vi "CheckVirtualSetup.vi"(8 "error in (no error)":errorcluster, 11 "VirtualDataTable":string[](array[string])) -> (0 "error out":errorcluster, 2 "VirtualNames":cluster{string[]}[](array[cluster]), 3 "VirtualSetups":string[](array[string]))   [LabVIEW 2014, in "Project.lvclass"]
uses:
  Project.lvclass
  VirtualSetupDataTypeDefine.ctl
  Virtual/Control/AllVirtualTypeData.ctl
  Virtual/VirtualOrigin.lvclass
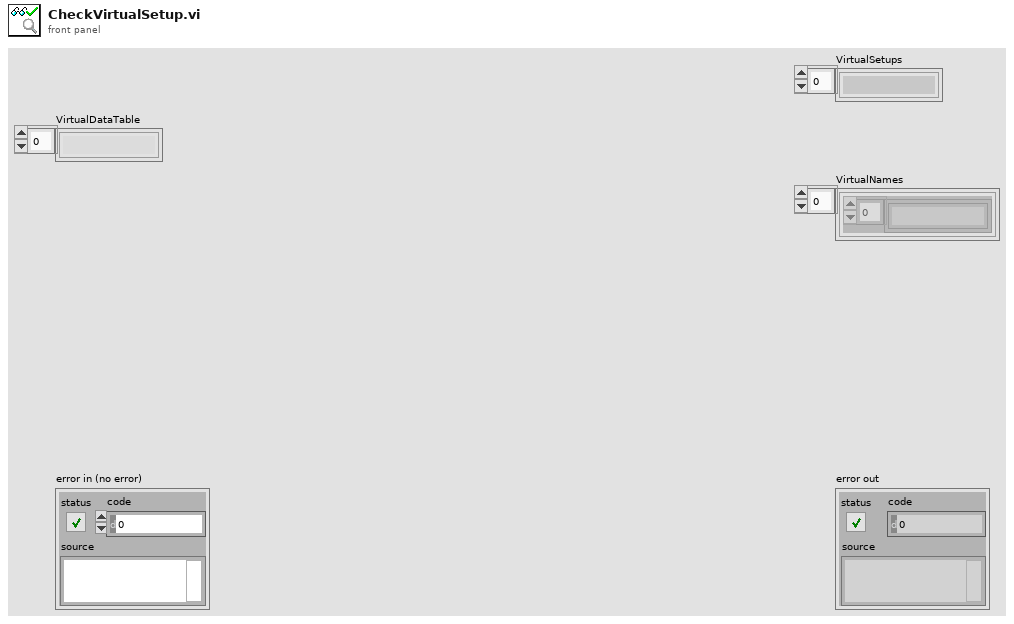
[diagram p1: front panel]
types:
  T1 = typedef "Project.lvclass/VirtualSetupDataTypeDefine.ctl" = T2[]
  T2 = typedef "VirtualOrigin.lvclass/AllVirtualTypeData.ctl" = cluster{"Search Name":string, "Start X":dbl, "Increase X":dbl, "X Step":i32, "Start Y":dbl, "Increase Y":dbl, "Y Step":i32, "Sensor":i32}
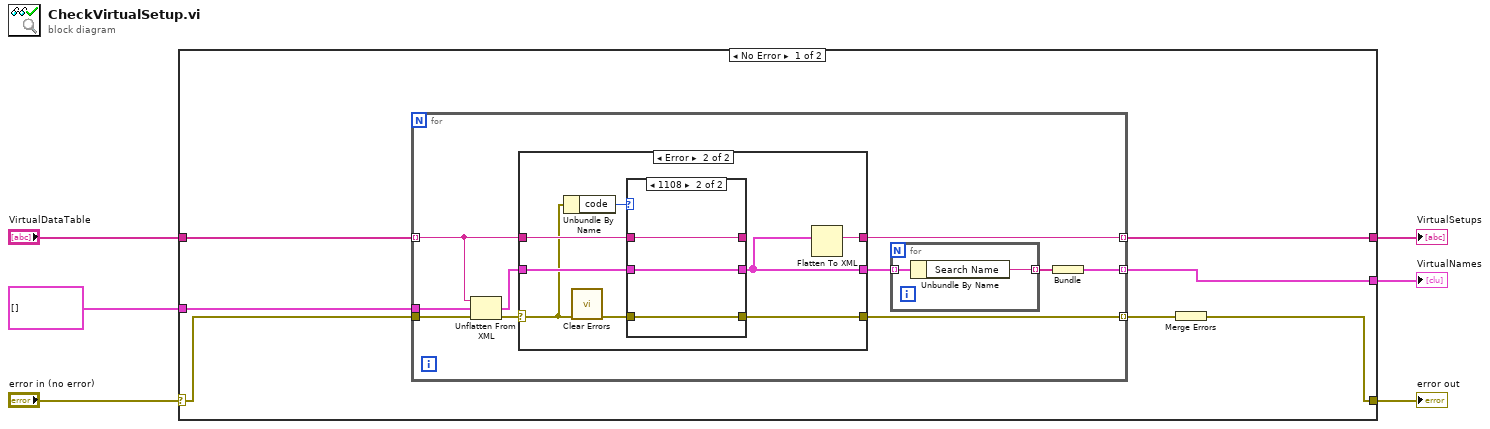
[diagram p0: block diagram]
diagram:
  n1 = case shown="No Error" "error in (no error)" {
    selector: "error in (no error)" -> [w13 w43]
    tunnel: [w11 w43] -> w5
    tunnel: [w10 _] -> w4
    tunnel: "VirtualDataTable" -> [w9 _]
    tunnel: [w8 _] -> w2
    tunnel: T1 [] ("VirtualSetupClusterArray") -> [w7 _]
    frame No Error {
      n2 = for {
        tunnel: w9 -> [w17] mode=indexing
        tunnel: w13 -> [w23]
        tunnel: [w20] -> w10 mode=indexing
        tunnel: w7 -> [w18]
        tunnel: [w16] -> w12 mode=indexing
        tunnel: [w14] -> w8 mode=indexing
        n3 = Unflatten From XML(xml string=w17, type=w18, error in (no error)=w23) -> (value=w21:T1, error out=w22:errorcluster)
        n4 = case shown="Error" w22 {
          selector: w22 -> [w28 w31]
          tunnel: w21 -> [w26 w35]
          tunnel: [w27 w30] -> w20
          tunnel: [w26 w29] -> w19
          tunnel: w17 -> [w27 w34]
          tunnel: [w28 w33] -> w16
          frame No Error {
          }
          frame Error {
            n5 = Unbundle By Name(w31) -> ("code"=w36:i32)
            n6 = call <vilib>:"Clear Errors.vi"("error in (no error)"=w31) -> ("error out"=w32:errorcluster)  [unwired: 5 in, 1 out]
            n7 = case shown="1108" w36 {
              tunnel: w32 -> [w38 w41]
              tunnel: w35 -> [w39 w42]
              tunnel: [w37 w40] -> _
              tunnel: [w39 w42] -> w29
              tunnel: w34 -> [w37 w40]
              tunnel: [w38 w41] -> w33
              frame Default {
              }
              frame 1108 {
              }
            }
            n8 = Flatten To XML(anything=w29) -> (xml string=w30:string)
          }
        }
        n9 = for {
          tunnel: w19 -> [w25] mode=indexing
          tunnel: [w24] -> w15 mode=indexing
          n10 = Unbundle By Name(w25) -> ("Search Name"=w24:string)
        }
        n11 = Bundle(w15) -> (w14:cluster{string[]})  [unwired: 1 in]
      }
      n12 = Merge Errors(w12) -> (w11:errorcluster)
    }
    frame Error {
    }
  }
  "error out" <- w5
  "VirtualSetups" <- w4
  "VirtualNames" <- w2
